vi "07_DoRegression_3el.vi"(10 "film H, nm":dbl=50.0, 11 "Input ChVoltage":T1) -> (0 "VoltageBelow, V":dbl, 2 "Regression":cluster{"VoltageRes, V":dbl, "Field, kV/cm":dbl}, 3 "PlotPoints":cluster{"Time":dbl[], "Voltage":dbl[]}(graph)={"Time"=[0.0, 0.00037111111108161925, 0.000510833333311085, 0.0006505555555405509, 0.0007766666666915019, 0.0009172222221968695, 0.0010569444444263353, 0.0011958333333152243, 0.0013350000000274223], "Voltage"=[5.89, 5.89, 5.89, 5.89, 5.89, 5.89, 5.89, 5.89, 5.89]})   [LabVIEW 2017]
uses:
  <vilib>/Analysis/6fits.llb/Curve Fitting Criteria.ctl
  <vilib>/Analysis/NI_AALPro.lvlib
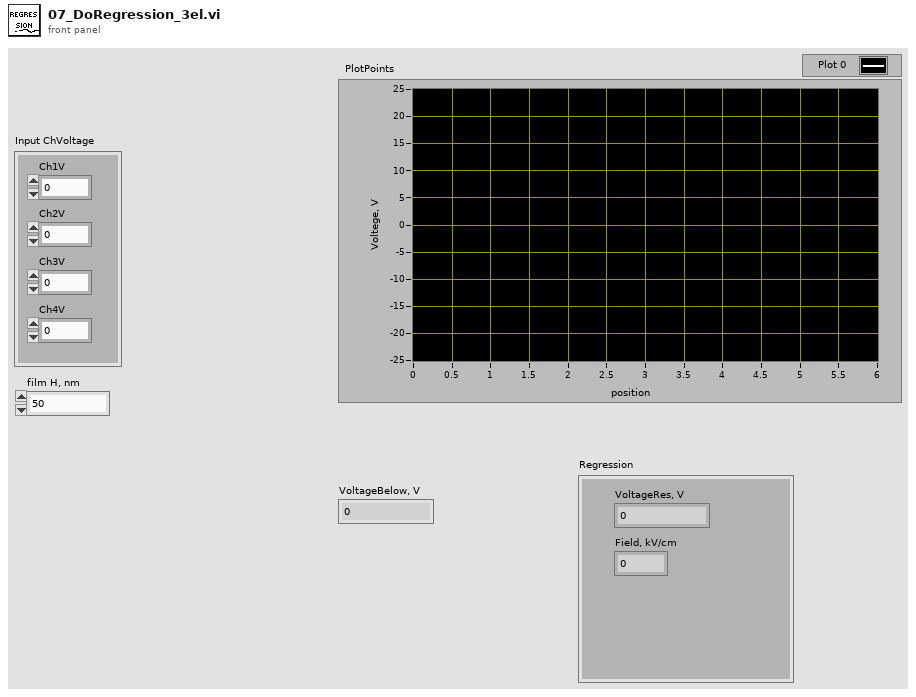
[diagram p1: front panel]
types:
  T1 = cluster{"Ch1V":dbl, "Ch2V":dbl, "Ch3V":dbl, "Ch4V":dbl}
  T2 = typedef "NI_AALPro.lvlib/Curve Fitting Criteria.ctl" = u16
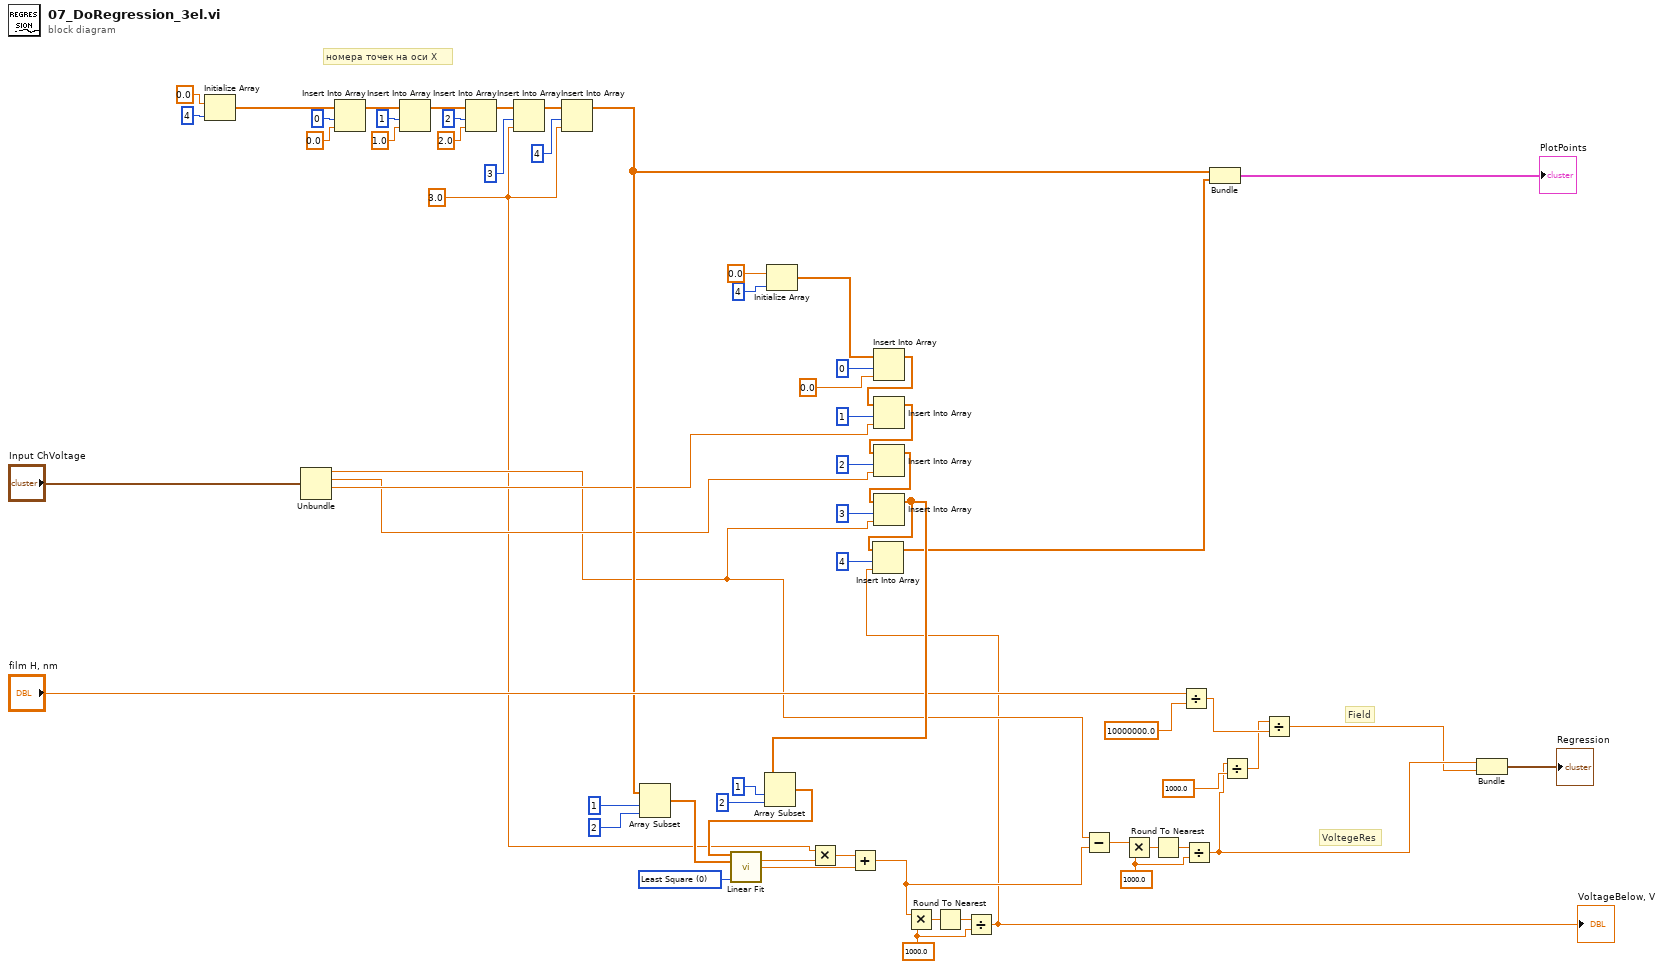
[diagram p0: block diagram]
diagram:
  w2 = 3.0 ("new element/subarray")
  w19 = 1000.0 ("y")
  w23 = 1000.0 ("y")
  w37 = T2 0 items=["Least Square", "Least Absolute Residual", "Bisquare"] ("method")
  # "Field"
  # "VoltegeRes"
  # "номера точек на оси X"
  n1 = Initialize Array(0.0 ("element"), 4 ("index")) -> (w1:dbl[])
  n2 = Unbundle("Input ChVoltage") -> ("Ch1V"=w5:dbl, "Ch2V"=w6:dbl, "Ch3V"=w7:dbl)  [unwired: 1 out]
  n3 = Insert Into Array(array=w1, index=0, new element=0.0 ("new element/subarray")) -> (w44:dbl[])
  n4 = Insert Into Array(array=w44, index=1, new element=1.0 ("new element/subarray")) -> (w43:dbl[])
  n5 = Insert Into Array(array=w43, index=2, new element=2.0 ("new element/subarray")) -> (w33:dbl[])
  n6 = Insert Into Array(array=w33, index=3, new element=w2) -> (w42:dbl[])
  n7 = Insert Into Array(array=w42, index=4, new element=w2) -> (w11:dbl[])
  n8 = Array Subset(array=w11, index=1, length=2) -> (w32:dbl[])
  n9 = Initialize Array(0.0 ("element"), 4 ("dimension size")) -> (w55:dbl[])
  n10 = Insert Into Array(array=w55, index=0, new element=0.0 ("new element/subarray")) -> (w41:dbl[])
  n11 = Insert Into Array(array=w41, index=1, new element=w7) -> (w40:dbl[])
  n12 = Insert Into Array(array=w40, index=2, new element=w6) -> (w38:dbl[])
  n13 = Insert Into Array(array=w38, index=3, new element=w5) -> (w29:dbl[])
  n14 = Array Subset(array=w29, index=1, length=2) -> (w28:dbl[])
  n15 = call <vilib>:"Linear Fit.vi"("Y"=w28, "X"=w32, "method"=w37) -> ("slope"=w35:dbl, "intercept"=w36:dbl)  [unwired: 8 in, 3 out]
  n16 = Multiply(x=w2, y=w35) -> (x*y=w34:dbl)
  n17 = Add(x=w34, y=w36) -> (x+y=w18:dbl)
  n18 = Multiply(x=w18, y=w19) -> (x*y=w21:dbl)
  n19 = Round To Nearest(number=w21) -> (nearest integer value=w20:dbl)
  n20 = Divide(x=w20, y=w19) -> (x/y=w3:dbl)
  "VoltageBelow, V" <- w3
  n21 = Insert Into Array(array=w29, index=4, new element=w3) -> (w4:dbl[])
  n22 = Subtract(x=w5, y=w18) -> (x-y=w22:dbl)
  n23 = Multiply(x=w22, y=w23) -> (x*y=w25:dbl)
  n24 = Round To Nearest(number=w25) -> (nearest integer value=w24:dbl)
  n25 = Divide(x="film H, nm", y=10000000.0) -> (x/y=w14:dbl)
  n26 = Divide(x=w24, y=w23) -> (x/y=w9:dbl)
  n27 = Bundle(w11, w4) -> (→"PlotPoints":cluster{dbl[], dbl[]})  [unwired: 1 in]
  n28 = Divide(x=w9, y=1000.0) -> (x/y=w13:dbl)
  n29 = Divide(x=w13, y=w14) -> (x/y=w8:dbl)
  n30 = Bundle(w9, w8) -> (→"Regression":cluster{dbl, dbl})  [unwired: 1 in]
